vi "GPS-Read.vi"(3 "Organised Output from the GPS":T1(tab)) -> ()   [LabVIEW 2019]
uses:
  <vilib>/Platform/TimedLoop/XDataNode/timing_clust.ctl
  <vilib>/Platform/TimedLoop/XDataNode/nitl_modes.ctl
  <vilib>/Platform/TimedLoop/XDataNode/wakeup.ctl
  <vilib>/Instr/_visa.llb/VISA Configure Serial Port (Instr).vi
  <vilib>/platform/TimedLoop/XDataNode/XDataNode.xnode
  <vilib>/Platform/TimedLoop/XDataNode/XDNodeRunTimeDep.lvlib
panel:
  out "Iteration Duration (ms)":i64
  out "GPGSV":string
  out "number of message":string
  out "msg1":string
  out "Satelite in view":string
  in  "Satelite_id/elevation/azimuth/SNR":enum32{"Msg 1", "Msg 2", "Msg 3", "Msg 4"}(tab)
  out "Satelite_id/elevation/azimuth/SNR":string[](array[string])
  out "Satelite_id/elevation/azimuth/SNR 2":string[](array[string])
  out "Satelite_id/elevation/azimuth/SNR 3":string[](array[string])
  out "Satelite_id/elevation/azimuth/SNR 4":string[](array[string])
  out "Signal ID / Check sum":string[](array[string])
  out "Signal ID / Check sum 2":string[](array[string])
  out "Satelite_id/elevation/azimuth/SNR 8":string[](array[string])
  out "Satelite_id/elevation/azimuth/SNR 7":string[](array[string])
  out "Satelite_id/elevation/azimuth/SNR 6":string[](array[string])
  out "Satelite_id/elevation/azimuth/SNR 5":string[](array[string])
  out "Signal ID / Check sum 3":string[](array[string])
  out "Satelite_id/elevation/azimuth/SNR 12":string[](array[string])
  out "Satelite_id/elevation/azimuth/SNR 11":string[](array[string])
  out "Satelite_id/elevation/azimuth/SNR 10":string[](array[string])
  out "Satelite_id/elevation/azimuth/SNR 9":string[](array[string])
  out "Signal ID / Check sum 4":string[](array[string])
  out "Satelite_id/elevation/azimuth/SNR 16":string[](array[string])
  out "Satelite_id/elevation/azimuth/SNR 15":string[](array[string])
  out "Satelite_id/elevation/azimuth/SNR 14":string[](array[string])
  out "Satelite_id/elevation/azimuth/SNR 13":string[](array[string])
  out "GLGSV 2":string
  out "number of message 2":string
  out "msg1 2":string
  out "Satelite in view 2":string
  in  "Satelite_id/elevation/azimuth/SNR":enum32{"Msg 1", "Msg 2", "Msg 3", "Msg 4"}(tab)
  out "Satelite_id/elevation/azimuth/SNR 20":string[](array[string])
  out "Satelite_id/elevation/azimuth/SNR 19":string[](array[string])
  out "Satelite_id/elevation/azimuth/SNR 18":string[](array[string])
  out "Satelite_id/elevation/azimuth/SNR 17":string[](array[string])
  out "Signal ID / Check sum 5":string[](array[string])
  out "Signal ID / Check sum 6":string[](array[string])
  out "Satelite_id/elevation/azimuth/SNR 21":string[](array[string])
  out "Satelite_id/elevation/azimuth/SNR 22":string[](array[string])
  out "Satelite_id/elevation/azimuth/SNR 23":string[](array[string])
  out "Satelite_id/elevation/azimuth/SNR 24":string[](array[string])
  out "Signal ID / Check sum 7":string[](array[string])
  out "Satelite_id/elevation/azimuth/SNR 25":string[](array[string])
  out "Satelite_id/elevation/azimuth/SNR 26":string[](array[string])
  out "Satelite_id/elevation/azimuth/SNR 27":string[](array[string])
  out "Satelite_id/elevation/azimuth/SNR 28":string[](array[string])
  out "Signal ID / Check sum 8":string[](array[string])
  out "Satelite_id/elevation/azimuth/SNR 29":string[](array[string])
  out "Satelite_id/elevation/azimuth/SNR 30":string[](array[string])
  out "Satelite_id/elevation/azimuth/SNR 31":string[](array[string])
  out "Satelite_id/elevation/azimuth/SNR 32":string[](array[string])
  out "GAGSV 3":string
  out "number of message 3":string
  out "msg1 3":string
  out "Satelite in view 3":string
  in  "Satelite_id/elevation/azimuth/SNR":enum32{"Msg 1", "Msg 2", "Msg 3", "Msg 4"}(tab)
  out "Satelite_id/elevation/azimuth/SNR 37":string[](array[string])
  out "Satelite_id/elevation/azimuth/SNR 36":string[](array[string])
  out "Satelite_id/elevation/azimuth/SNR 35":string[](array[string])
  out "Satelite_id/elevation/azimuth/SNR 34":string[](array[string])
  out "Signal ID / Check sum 9":string[](array[string])
  out "Signal ID / Check sum 10":string[](array[string])
  out "Satelite_id/elevation/azimuth/SNR 38":string[](array[string])
  out "Satelite_id/elevation/azimuth/SNR 39":string[](array[string])
  out "Satelite_id/elevation/azimuth/SNR 40":string[](array[string])
  out "Satelite_id/elevation/azimuth/SNR 41":string[](array[string])
  out "Signal ID / Check sum 11":string[](array[string])
  out "Satelite_id/elevation/azimuth/SNR 42":string[](array[string])
  out "Satelite_id/elevation/azimuth/SNR 43":string[](array[string])
  out "Satelite_id/elevation/azimuth/SNR 44":string[](array[string])
  out "Satelite_id/elevation/azimuth/SNR 45":string[](array[string])
  out "Signal ID / Check sum 12":string[](array[string])
  out "Satelite_id/elevation/azimuth/SNR 46":string[](array[string])
  out "Satelite_id/elevation/azimuth/SNR 47":string[](array[string])
  out "Satelite_id/elevation/azimuth/SNR 48":string[](array[string])
  out "Satelite_id/elevation/azimuth/SNR 49":string[](array[string])
  out "GBGSV 4":string
  out "number of message 4":string
  out "msg1 4":string
  out "Satelite in view 4":string
  in  "Satelite_id/elevation/azimuth/SNR":enum32{"Msg 1", "Msg 2", "Msg 3", "Msg 4"}(tab)
  out "Satelite_id/elevation/azimuth/SNR 54":string[](array[string])
  out "Satelite_id/elevation/azimuth/SNR 53":string[](array[string])
  out "Satelite_id/elevation/azimuth/SNR 52":string[](array[string])
  out "Satelite_id/elevation/azimuth/SNR 51":string[](array[string])
  out "Signal ID / Check sum 13":string[](array[string])
  out "Signal ID / Check sum 14":string[](array[string])
  out "Satelite_id/elevation/azimuth/SNR 55":string[](array[string])
  out "Satelite_id/elevation/azimuth/SNR 56":string[](array[string])
  out "Satelite_id/elevation/azimuth/SNR 57":string[](array[string])
  out "Satelite_id/elevation/azimuth/SNR 58":string[](array[string])
  out "Signal ID / Check sum 15":string[](array[string])
  out "Satelite_id/elevation/azimuth/SNR 59":string[](array[string])
  out "Satelite_id/elevation/azimuth/SNR 60":string[](array[string])
  out "Satelite_id/elevation/azimuth/SNR 61":string[](array[string])
  out "Satelite_id/elevation/azimuth/SNR 62":string[](array[string])
  out "Signal ID / Check sum 16":string[](array[string])
  out "Satelite_id/elevation/azimuth/SNR 63":string[](array[string])
  out "Satelite_id/elevation/azimuth/SNR 64":string[](array[string])
  out "Satelite_id/elevation/azimuth/SNR 65":string[](array[string])
  out "Satelite_id/elevation/azimuth/SNR 66":string[](array[string])
  out "UTC Time":string
  out "N/S":string
  out "Long":string
  out "Mode":string
  out "Status":string
  out "Lat":string
  out "Course over Ground [Degrees]":string
  out "date[ddmmyy]":string
  out "E/W":string
  out "Speed over ground[knot]":string
  out "xxRMC":string
  out "NavStatus":string
  out "Checksum":string
  out "Carriage return":string
  out "Lat":string
  out "NS":string
  out "GLL":string
  out "Long 3":string
  out "EW":string
  out "Time":string
  out "Status 2":string
  out "Positioning mod":string
  out "Check sum":string
  out "Carriage return 2":string
  out "VTG":string
  out "Course over Ground":string
  out "Reference":string
  out "Course over Ground (Magnetic)":string
  out "Reference2":string
  out "Speedover Ground (knots)":string
  out "Units1":string
  out "Speed over ground kph":string
  out "Units 2":string
  out "Position Mode 2":string
  out "Check sum":string
  out "GGA 3":string
  out "UTC time":string
  out "Lat 2":string
  out "NS":string
  out "Long 2":string
  out "EW":string
  out "Pos_indicator":string
  out "Number of Satelite_used":string
  out "hdop":string
  out "msl_altitude":string
  out "altitude_units":string
  out "geoidal_Seperation":string
  out "Separation unit":string
  out "age of Diff corr":string
  out "diffStating":string
  out "Checksum":string
  out "GSA":string
  out "Operation Mode":string
  out "Navigation mode":string
  out "satelite used channel 1":string
  out "satelite used channel 3":string
  out "satelite used channel 4":string
  out "satelite used channel 5":string
  out "satelite used channel 6":string
  out "satelite used channel 7":string
  out "satelite used channel 8":string
  out "satelite used channel 9":string
  out "satelite used channel 10":string
  out "satelite used channel 11":string
  out "satelite used channel 12":string
  out "pdop":string
  out "hdop 2":string
  out "vdop":string
  out "System ID":string
  out "Checksum":string
  out "satelite used channel 2":string
  out "Raw output from GPS":string
  in  "stop":bool
  # "Signal ID / Check sum"
  # "Signal ID / Check sum"
  # "Signal ID / Check sum"
  # "Signal ID / Check sum"
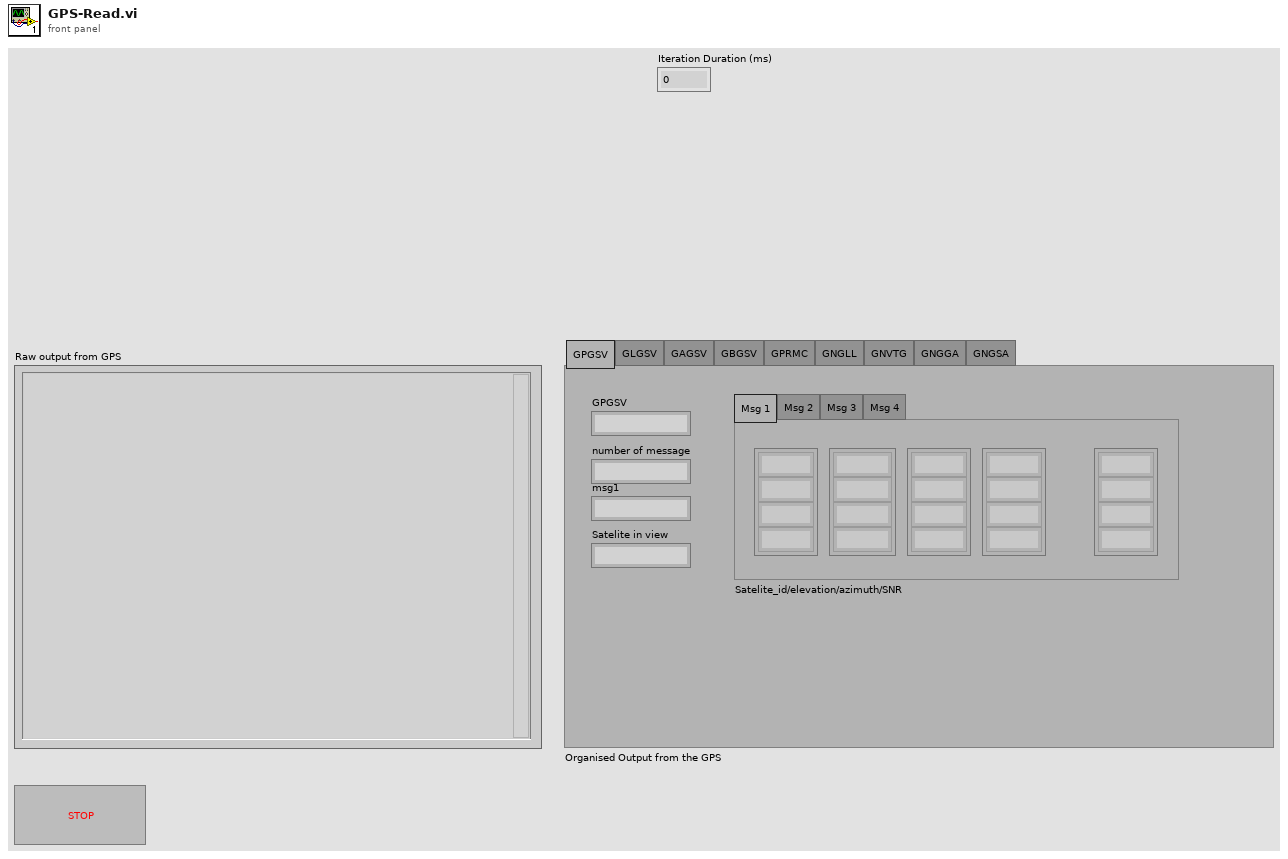
[diagram p1: front panel]
types:
  T1 = enum32{"GPGSV", "GLGSV", "GAGSV", "GBGSV", "GPRMC", "GNGLL", "GNVTG", "GNGGA", "GNGSA"}
  T2 = typedef "XDNodeRunTimeDep.lvlib/timing_clust.ctl" = cluster{"Expected End [f-1]":u64, "Actual End [f-1]":u64, "Finished Late? [f-1]":bool, "Expected End [i-1]":u64, "Actual End [i-1]":u64, "Finished Late? [i-1]":bool, "Expected Start [i]":u64, "Actual Start [i]":u64, "Expected Start [f]":u64, "Actual Start [f]":u64, "Source Name":string, "Structure Name":string, "Period":i64, "Deadline":i64, "Offset":i64, "Start":i64, "Priority":i32, "Timeout":i32, "Mode":T3, "Wakeup Reason":T4, "Error":errorcluster, "Source Type":string, "Secondary Source Type":string, "Global End Time":u64, "Global Start Time":u64, "Frame Duration":u64, "Iteration Duration":u64, "Assigned CPU":i32, "I/O Scan Engine Mode":u32}
  T3 = typedef "XDNodeRunTimeDep.lvlib/nitl_modes.ctl" = enum32{"No Change", "Process missed periods, maintain original phase", "Discard missed periods, maintain original phase", "Process missed periods, ignore original phase", "Discard missed periods, ignore original phase"}
  T4 = typedef "XDNodeRunTimeDep.lvlib/wakeup.ctl" = enum32{"Normal", "Aborted", "Asynchronous wakeup", "Timing source error", "Timed loop error", "Timeout"}
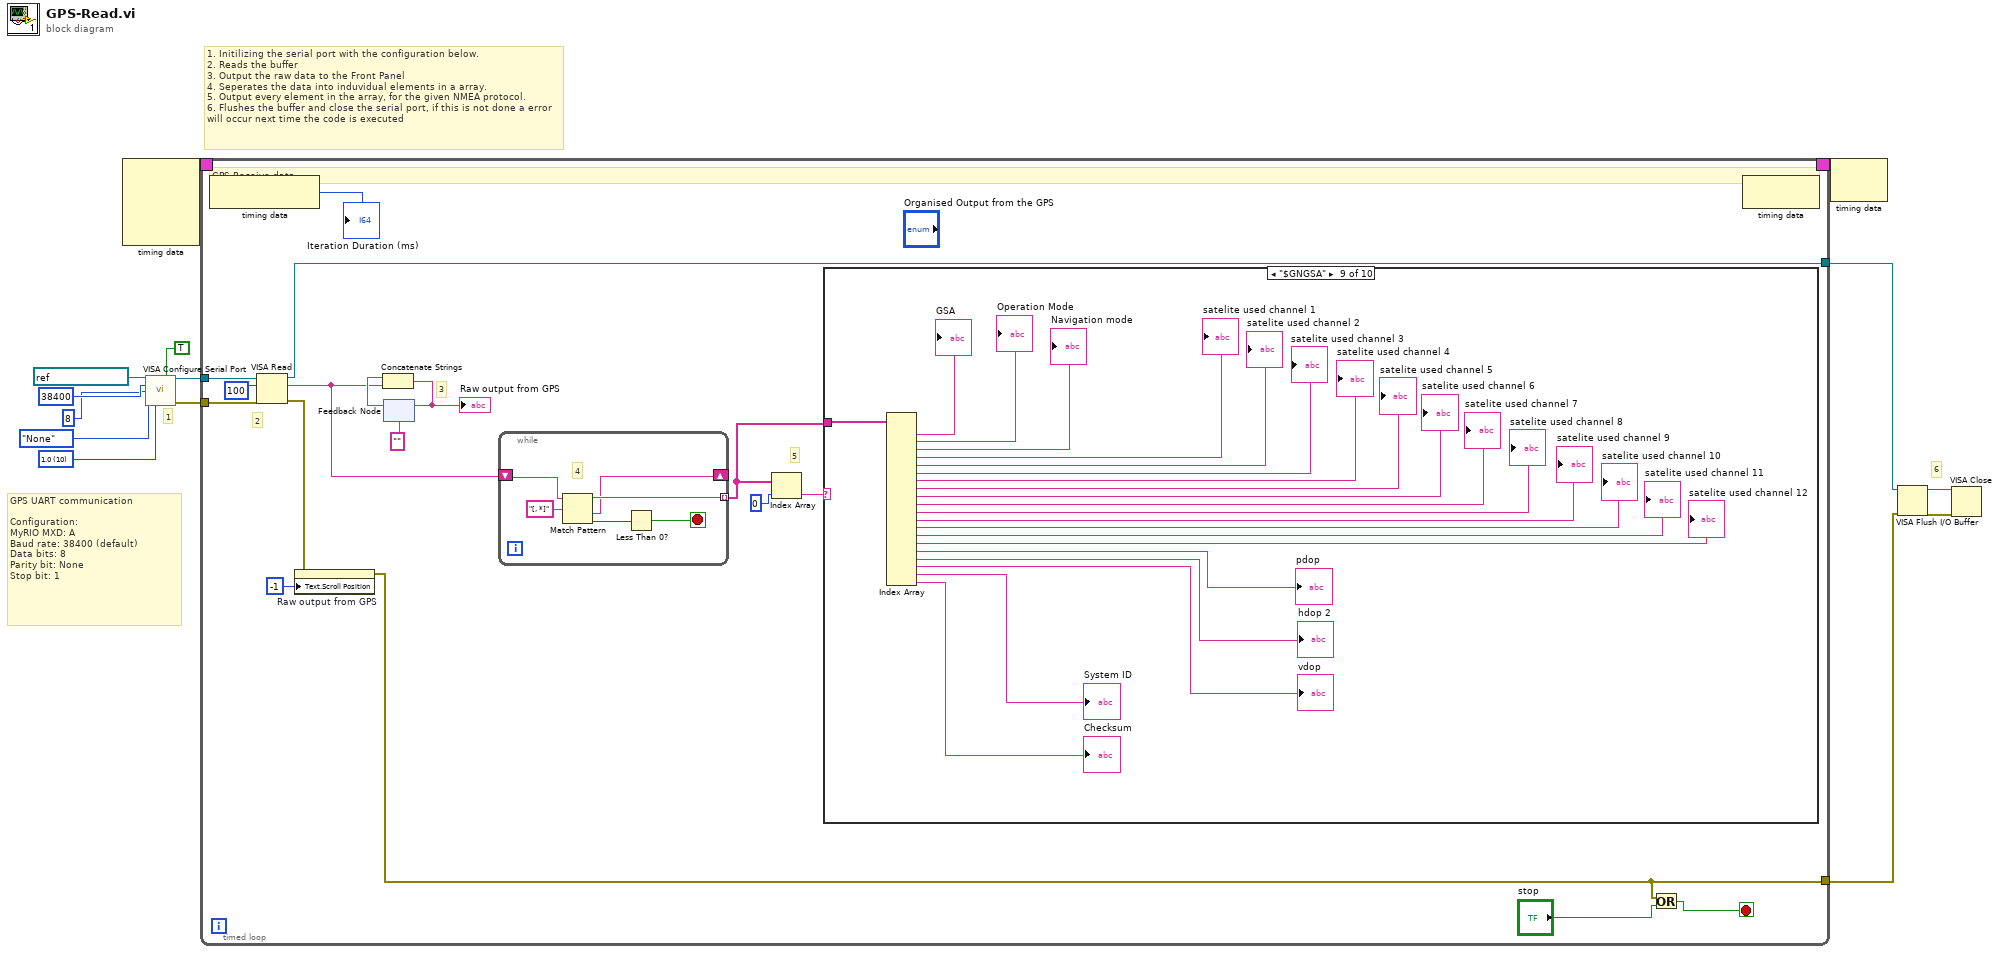
[diagram p0: block diagram]
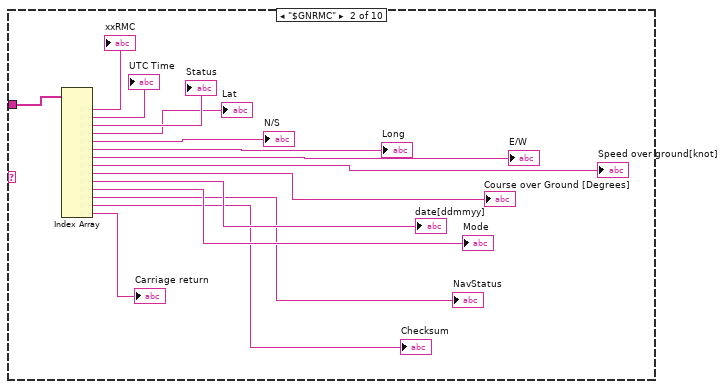
[diagram p3: hidden frame]
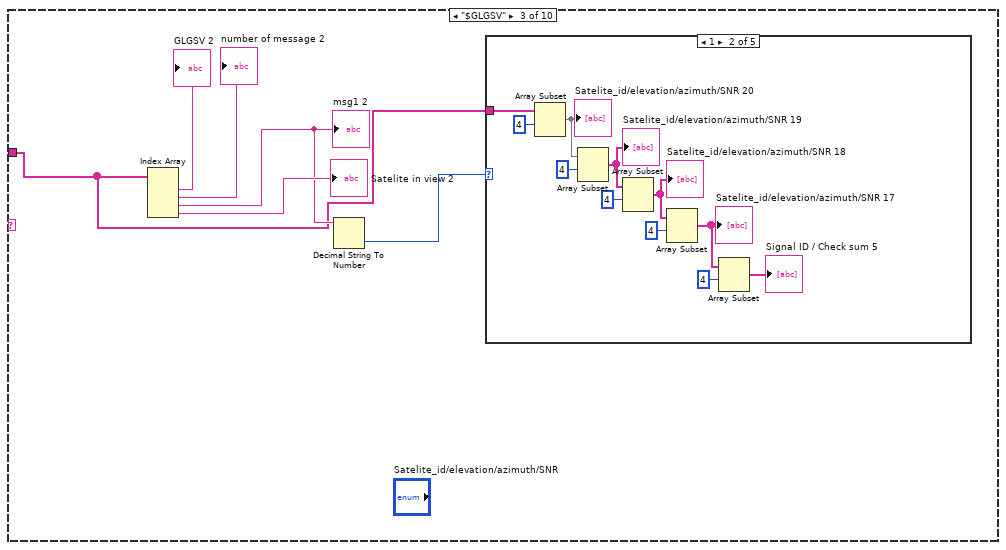
[diagram p4: hidden frame]
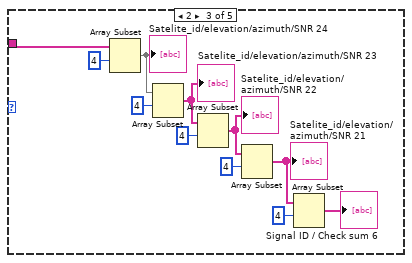
[diagram p6: hidden frame]
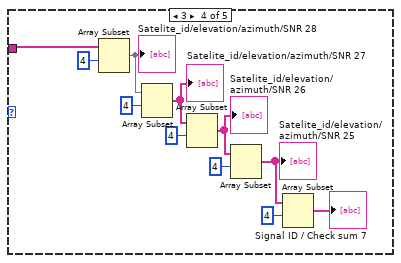
[diagram p7: hidden frame]
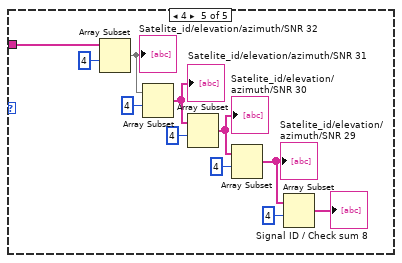
[diagram p8: hidden frame]
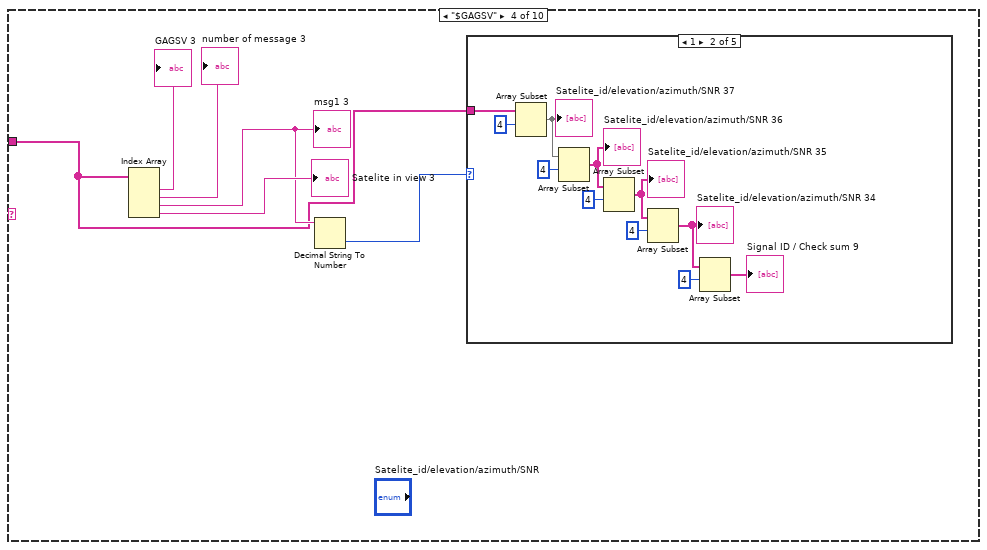
[diagram p9: hidden frame]
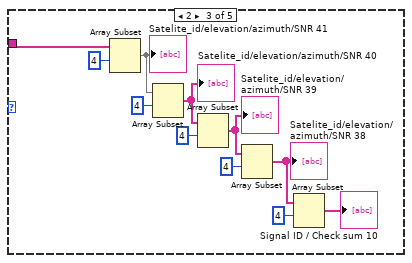
[diagram p11: hidden frame]
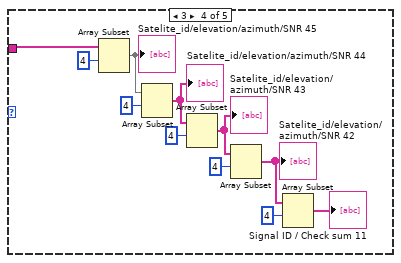
[diagram p12: hidden frame]
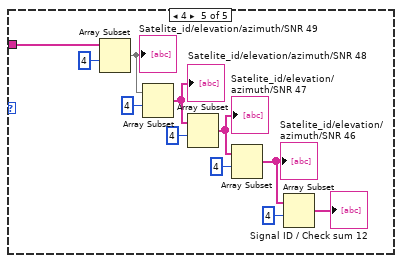
[diagram p13: hidden frame]
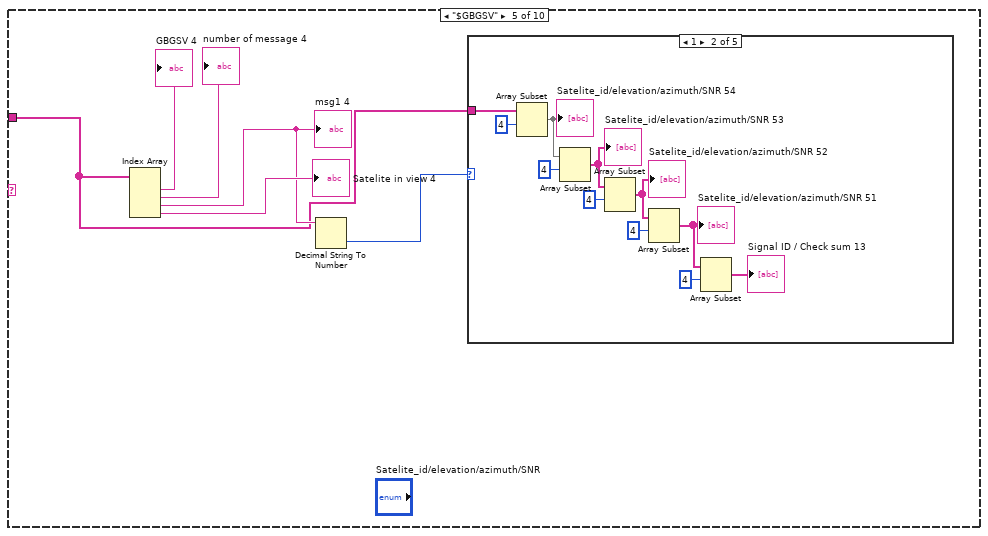
[diagram p14: hidden frame]
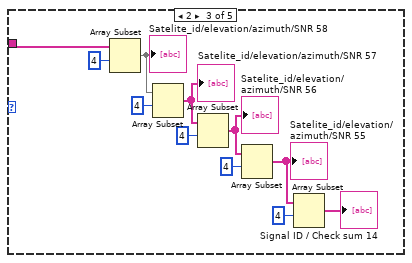
[diagram p16: hidden frame]
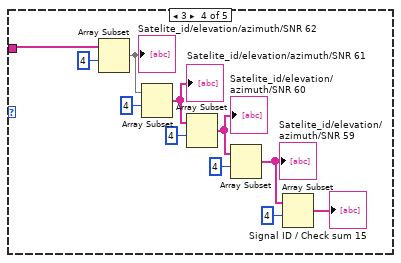
[diagram p17: hidden frame]
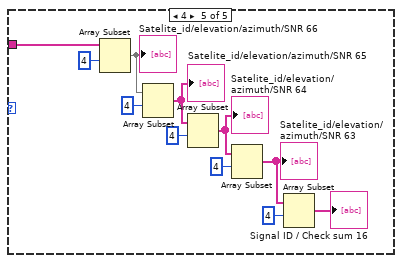
[diagram p18: hidden frame]
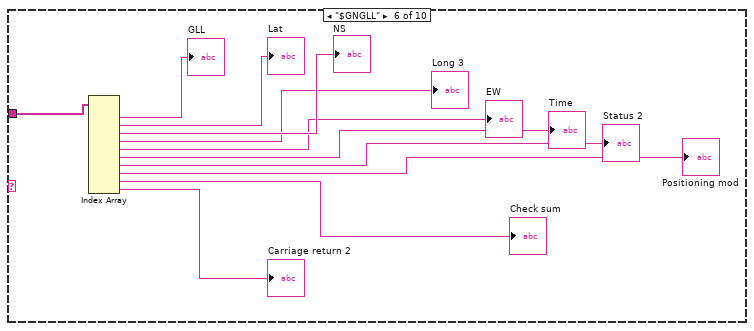
[diagram p19: hidden frame]
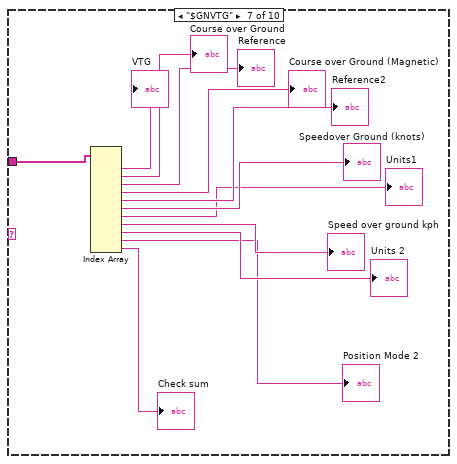
[diagram p20: hidden frame]
diagram:
  w9 = u16 10 items=["1.0"=10, "1.5"=15, "2.0"=20] ("stop bits (10: 1 bit)")
  # "6"
  # "1"
  # "1. Initilizing the serial port with the configuration below.\n2. Reads the buffer\n3. Output the raw data to the Front Panel\n4. Seperates the data into induvidual elements in a array.\n5. Output every element in the array, for the given NMEA protocol.\n6. Flushes the buffer and close the serial port, if this is not done a error will occur next time the code is executed"
  # "GPS UART communication\n\nConfiguration:\nMyRIO MXD: A\nBaud rate: 38400 (default)\nData bits: 8\nParity bit: None\nStop bit: 1"
  n1 = node-c288() -> (w2:T2)  [unwired: 4 in]
  n2 = call-poly "VISA Configure Serial Port"("VISA resource name"=refnum<visa-resource-name> "ASRL1::INSTR", "Enable Termination\nChar (T)"=TRUE ("Enable Termination\nChar (T)"), "baud rate (9600)"=u32 38400, "data bits (8)"=u16 8, "parity (0:none)"=enum16{"None", "Odd", "Even", "Mark", "Space"}."None", "stop bits (10: 1 bit)"=w9) -> ("VISA resource name out"=w5:refnum<visa-resource-name>, "error out"=w4:errorcluster)  [unwired: 8 in]
  n3 = timed-loop {
    tunnel: [w23] -> w6
    tunnel: w5 -> [w22]
    tunnel: w4 -> [w21]
    tunnel: [w17] -> w3
    timing: w2 -> [_]
    timing-out: [_] -> w1
    stop <- w20 stop-if-true
    # "5"
    # "3"
    # "2"
    # "GPS Receive data"
    n4 = node-c288() -> (→"Iteration Duration (ms)":i64)  [unwired: 1 in]
    n5 = VISA Read(VISA resource name=w22, byte count=u32 100, error in (no error)=w21) -> (VISA resource name out=w23:refnum<visa-resource-name>, read buffer=w27:string, error out=w18:errorcluster)  [unwired: 1 out]
    n6 = property on="Raw output from GPS" class="Str"(error in=w18, "Text.Scroll Position"=-1 ("Label.Scroll Position")) -> (error out=w17:errorcluster)  [unwired: 1 in, 1 out]
    n7 = feedback #1("") -> (w29:string)
    n8 = Concatenate Strings(w29, w27) -> (w30:string)
    "Raw output from GPS" <- w30
    n9 = feedback-in #1(w30) -> ()
    n10 = while {
      tunnel: [w314] -> w24 mode=indexing
      shift-right: [w313] -> _
      shift-left: w27 -> [w316]
      stop <- w311 stop-if-true
      # "4"
      n11 = Match Pattern(string=w316, regular expression="[, *]") -> (before substring=w314:string, after substring=w313:string, offset past match=w312:i32)  [unwired: 1 in, 1 out]
      n12 = Less Than 0?(x=w312) -> (x < 0?=w311:bool)
    }
    n13 = Index Array(array=w24, index=0) -> (element=w25:string)
    n14 = case shown="\"$GNGSA\"" w25 {
      tunnel: w24 -> [_ w49 w50 w100 w150 w210 w222 w239 w260 w261]
      frame "False", Default {
      }
      frame "$GNRMC" {
        n15 = Index Array(array=w49) -> (element #1=→"xxRMC":string, element #2=→"UTC Time":string, element #3=→"Status":string, element #4=→"Lat":string, element #5=→"N/S":string, element #6=→"Long":string, element #7=→"E/W":string, element #8=→"Speed over ground[knot]":string, element #9=→"Course over Ground [Degrees]":string, element #10=→"date[ddmmyy]":string, element #11=→"Mode":string, element #12=→"NavStatus":string, element #13=→"Checksum":string, element #14=→"Carriage return":string)  [unwired: 14 in]
      }
      frame "$GLGSV" {
        n16 = Index Array(array=w50) -> (element #1=→"GLGSV 2":string, element #2=→"number of message 2":string, element #3=w52:string, element #4=→"Satelite in view 2":string)  [unwired: 4 in]
        "msg1 2" <- w52
        n17 = Decimal String To Number(string=w52) -> (number=w51:i32)  [unwired: 2 in, 1 out]
        n18 = case shown="1" w51 {
          tunnel: w50 -> [_ w57 w67 w78 w89]
          frame 0, Default {
          }
          frame 1 {
            n19 = Array Subset(array=w57, index=4) -> (w62:string[])  [unwired: 1 in]
            "Satelite_id/elevation/azimuth/SNR 20" <- w62
            n20 = Array Subset(array=w62, index=4) -> (w63:string[])  [unwired: 1 in]
            "Satelite_id/elevation/azimuth/SNR 19" <- w63
            n21 = Array Subset(array=w63, index=4) -> (w64:string[])  [unwired: 1 in]
            "Satelite_id/elevation/azimuth/SNR 18" <- w64
            n22 = Array Subset(array=w64, index=4) -> (w66:string[])  [unwired: 1 in]
            "Satelite_id/elevation/azimuth/SNR 17" <- w66
            n23 = Array Subset(array=w66, index=4) -> (→"Signal ID / Check sum 5":string[])  [unwired: 1 in]
          }
          frame 2 {
            n24 = Array Subset(array=w67, index=4) -> (w73:string[])  [unwired: 1 in]
            "Satelite_id/elevation/azimuth/SNR 24" <- w73
            n25 = Array Subset(array=w73, index=4) -> (w74:string[])  [unwired: 1 in]
            "Satelite_id/elevation/azimuth/SNR 23" <- w74
            n26 = Array Subset(array=w74, index=4) -> (w75:string[])  [unwired: 1 in]
            "Satelite_id/elevation/azimuth/SNR 22" <- w75
            n27 = Array Subset(array=w75, index=4) -> (w77:string[])  [unwired: 1 in]
            "Satelite_id/elevation/azimuth/SNR 21" <- w77
            n28 = Array Subset(array=w77, index=4) -> (→"Signal ID / Check sum 6":string[])  [unwired: 1 in]
          }
          frame 3 {
            n29 = Array Subset(array=w78, index=4) -> (w84:string[])  [unwired: 1 in]
            "Satelite_id/elevation/azimuth/SNR 28" <- w84
            n30 = Array Subset(array=w84, index=4) -> (w85:string[])  [unwired: 1 in]
            "Satelite_id/elevation/azimuth/SNR 27" <- w85
            n31 = Array Subset(array=w85, index=4) -> (w86:string[])  [unwired: 1 in]
            "Satelite_id/elevation/azimuth/SNR 26" <- w86
            n32 = Array Subset(array=w86, index=4) -> (w88:string[])  [unwired: 1 in]
            "Satelite_id/elevation/azimuth/SNR 25" <- w88
            n33 = Array Subset(array=w88, index=4) -> (→"Signal ID / Check sum 7":string[])  [unwired: 1 in]
          }
          frame 4 {
            n34 = Array Subset(array=w89, index=4) -> (w95:string[])  [unwired: 1 in]
            "Satelite_id/elevation/azimuth/SNR 32" <- w95
            n35 = Array Subset(array=w95, index=4) -> (w96:string[])  [unwired: 1 in]
            "Satelite_id/elevation/azimuth/SNR 31" <- w96
            n36 = Array Subset(array=w96, index=4) -> (w97:string[])  [unwired: 1 in]
            "Satelite_id/elevation/azimuth/SNR 30" <- w97
            n37 = Array Subset(array=w97, index=4) -> (w99:string[])  [unwired: 1 in]
            "Satelite_id/elevation/azimuth/SNR 29" <- w99
            n38 = Array Subset(array=w99, index=4) -> (→"Signal ID / Check sum 8":string[])  [unwired: 1 in]
          }
        }
      }
      frame "$GAGSV" {
        n39 = Index Array(array=w100) -> (element #1=→"GAGSV 3":string, element #2=→"number of message 3":string, element #3=w102:string, element #4=→"Satelite in view 3":string)  [unwired: 4 in]
        "msg1 3" <- w102
        n40 = Decimal String To Number(string=w102) -> (number=w101:i32)  [unwired: 2 in, 1 out]
        n41 = case shown="1" w101 {
          tunnel: w100 -> [_ w107 w117 w128 w139]
          frame 0, Default {
          }
          frame 1 {
            n42 = Array Subset(array=w107, index=4) -> (w112:string[])  [unwired: 1 in]
            "Satelite_id/elevation/azimuth/SNR 37" <- w112
            n43 = Array Subset(array=w112, index=4) -> (w113:string[])  [unwired: 1 in]
            "Satelite_id/elevation/azimuth/SNR 36" <- w113
            n44 = Array Subset(array=w113, index=4) -> (w114:string[])  [unwired: 1 in]
            "Satelite_id/elevation/azimuth/SNR 35" <- w114
            n45 = Array Subset(array=w114, index=4) -> (w116:string[])  [unwired: 1 in]
            "Satelite_id/elevation/azimuth/SNR 34" <- w116
            n46 = Array Subset(array=w116, index=4) -> (→"Signal ID / Check sum 9":string[])  [unwired: 1 in]
          }
          frame 2 {
            n47 = Array Subset(array=w117, index=4) -> (w123:string[])  [unwired: 1 in]
            "Satelite_id/elevation/azimuth/SNR 41" <- w123
            n48 = Array Subset(array=w123, index=4) -> (w124:string[])  [unwired: 1 in]
            "Satelite_id/elevation/azimuth/SNR 40" <- w124
            n49 = Array Subset(array=w124, index=4) -> (w125:string[])  [unwired: 1 in]
            "Satelite_id/elevation/azimuth/SNR 39" <- w125
            n50 = Array Subset(array=w125, index=4) -> (w127:string[])  [unwired: 1 in]
            "Satelite_id/elevation/azimuth/SNR 38" <- w127
            n51 = Array Subset(array=w127, index=4) -> (→"Signal ID / Check sum 10":string[])  [unwired: 1 in]
          }
          frame 3 {
            n52 = Array Subset(array=w128, index=4) -> (w134:string[])  [unwired: 1 in]
            "Satelite_id/elevation/azimuth/SNR 45" <- w134
            n53 = Array Subset(array=w134, index=4) -> (w135:string[])  [unwired: 1 in]
            "Satelite_id/elevation/azimuth/SNR 44" <- w135
            n54 = Array Subset(array=w135, index=4) -> (w136:string[])  [unwired: 1 in]
            "Satelite_id/elevation/azimuth/SNR 43" <- w136
            n55 = Array Subset(array=w136, index=4) -> (w138:string[])  [unwired: 1 in]
            "Satelite_id/elevation/azimuth/SNR 42" <- w138
            n56 = Array Subset(array=w138, index=4) -> (→"Signal ID / Check sum 11":string[])  [unwired: 1 in]
          }
          frame 4 {
            n57 = Array Subset(array=w139, index=4) -> (w145:string[])  [unwired: 1 in]
            "Satelite_id/elevation/azimuth/SNR 49" <- w145
            n58 = Array Subset(array=w145, index=4) -> (w146:string[])  [unwired: 1 in]
            "Satelite_id/elevation/azimuth/SNR 48" <- w146
            n59 = Array Subset(array=w146, index=4) -> (w147:string[])  [unwired: 1 in]
            "Satelite_id/elevation/azimuth/SNR 47" <- w147
            n60 = Array Subset(array=w147, index=4) -> (w149:string[])  [unwired: 1 in]
            "Satelite_id/elevation/azimuth/SNR 46" <- w149
            n61 = Array Subset(array=w149, index=4) -> (→"Signal ID / Check sum 12":string[])  [unwired: 1 in]
          }
        }
      }
      frame "$GBGSV" {
        n62 = Index Array(array=w150) -> (element #1=→"GBGSV 4":string, element #2=→"number of message 4":string, element #3=w152:string, element #4=→"Satelite in view 4":string)  [unwired: 4 in]
        "msg1 4" <- w152
        n63 = Decimal String To Number(string=w152) -> (number=w151:i32)  [unwired: 2 in, 1 out]
        n64 = case shown="1" w151 {
          tunnel: w150 -> [_ w157 w167 w178 w189]
          frame 0, Default {
          }
          frame 1 {
            n65 = Array Subset(array=w157, index=4) -> (w162:string[])  [unwired: 1 in]
            "Satelite_id/elevation/azimuth/SNR 54" <- w162
            n66 = Array Subset(array=w162, index=4) -> (w163:string[])  [unwired: 1 in]
            "Satelite_id/elevation/azimuth/SNR 53" <- w163
            n67 = Array Subset(array=w163, index=4) -> (w164:string[])  [unwired: 1 in]
            "Satelite_id/elevation/azimuth/SNR 52" <- w164
            n68 = Array Subset(array=w164, index=4) -> (w166:string[])  [unwired: 1 in]
            "Satelite_id/elevation/azimuth/SNR 51" <- w166
            n69 = Array Subset(array=w166, index=4) -> (→"Signal ID / Check sum 13":string[])  [unwired: 1 in]
          }
          frame 2 {
            n70 = Array Subset(array=w167, index=4) -> (w173:string[])  [unwired: 1 in]
            "Satelite_id/elevation/azimuth/SNR 58" <- w173
            n71 = Array Subset(array=w173, index=4) -> (w174:string[])  [unwired: 1 in]
            "Satelite_id/elevation/azimuth/SNR 57" <- w174
            n72 = Array Subset(array=w174, index=4) -> (w175:string[])  [unwired: 1 in]
            "Satelite_id/elevation/azimuth/SNR 56" <- w175
            n73 = Array Subset(array=w175, index=4) -> (w177:string[])  [unwired: 1 in]
            "Satelite_id/elevation/azimuth/SNR 55" <- w177
            n74 = Array Subset(array=w177, index=4) -> (→"Signal ID / Check sum 14":string[])  [unwired: 1 in]
          }
          frame 3 {
            n75 = Array Subset(array=w178, index=4) -> (w184:string[])  [unwired: 1 in]
            "Satelite_id/elevation/azimuth/SNR 62" <- w184
            n76 = Array Subset(array=w184, index=4) -> (w185:string[])  [unwired: 1 in]
            "Satelite_id/elevation/azimuth/SNR 61" <- w185
            n77 = Array Subset(array=w185, index=4) -> (w186:string[])  [unwired: 1 in]
            "Satelite_id/elevation/azimuth/SNR 60" <- w186
            n78 = Array Subset(array=w186, index=4) -> (w188:string[])  [unwired: 1 in]
            "Satelite_id/elevation/azimuth/SNR 59" <- w188
            n79 = Array Subset(array=w188, index=4) -> (→"Signal ID / Check sum 15":string[])  [unwired: 1 in]
          }
          frame 4 {
            n80 = Array Subset(array=w189, index=4) -> (w195:string[])  [unwired: 1 in]
            "Satelite_id/elevation/azimuth/SNR 66" <- w195
            n81 = Array Subset(array=w195, index=4) -> (w196:string[])  [unwired: 1 in]
            "Satelite_id/elevation/azimuth/SNR 65" <- w196
            n82 = Array Subset(array=w196, index=4) -> (w197:string[])  [unwired: 1 in]
            "Satelite_id/elevation/azimuth/SNR 64" <- w197
            n83 = Array Subset(array=w197, index=4) -> (w199:string[])  [unwired: 1 in]
            "Satelite_id/elevation/azimuth/SNR 63" <- w199
            n84 = Array Subset(array=w199, index=4) -> (→"Signal ID / Check sum 16":string[])  [unwired: 1 in]
          }
        }
      }
      frame "$GNGLL" {
        n85 = Index Array(array=w210) -> (element #1=→"GLL":string, element #2=→"Lat":string, element #3=→"NS":string, element #4=→"Long 3":string, element #5=→"EW":string, element #6=→"Time":string, element #7=→"Status 2":string, element #8=→"Positioning mod":string, element #9=→"Check sum":string, element #10=→"Carriage return 2":string)  [unwired: 10 in]
      }
      frame "$GNVTG" {
        n86 = Index Array(array=w222) -> (element #1=→"VTG":string, element #2=→"Course over Ground":string, element #3=→"Reference":string, element #4=→"Course over Ground (Magnetic)":string, element #5=→"Reference2":string, element #6=→"Speedover Ground (knots)":string, element #7=→"Units1":string, element #8=→"Speed over ground kph":string, element #9=→"Units 2":string, element #10=→"Position Mode 2":string, element #11=→"Check sum":string)  [unwired: 11 in]
      }
      frame "$GNGGA" {
        n87 = Index Array(array=w239) -> (element #1=→"GGA 3":string, element #2=→"UTC time":string, element #3=→"Lat 2":string, element #4=→"NS":string, element #5=→"Long 2":string, element #6=→"EW":string, element #7=→"Pos_indicator":string, element #8=→"Number of Satelite_used":string, element #9=→"hdop":string, element #10=→"msl_altitude":string, element #11=→"altitude_units":string, element #12=→"geoidal_Seperation":string, element #13=→"Separation unit":string, element #14=→"age of Diff corr":string, element #15=→"diffStating":string, element #16=→"Checksum":string)  [unwired: 16 in]
      }
      frame "$GNGSA" {
        n88 = Index Array(array=w260) -> (element #1=→"GSA":string, element #2=→"Operation Mode":string, element #3=→"Navigation mode":string, element #4=→"satelite used channel 1":string, element #5=→"satelite used channel 2":string, element #6=→"satelite used channel 3":string, element #7=→"satelite used channel 4":string, element #8=→"satelite used channel 5":string, element #9=→"satelite used channel 6":string, element #10=→"satelite used channel 7":string, element #11=→"satelite used channel 8":string, element #12=→"satelite used channel 9":string, element #13=→"satelite used channel 10":string, element #14=→"satelite used channel 11":string, element #15=→"satelite used channel 12":string, element #16=→"pdop":string, element #17=→"hdop 2":string, element #18=→"vdop":string, element #19=→"System ID":string, element #20=→"Checksum":string)  [unwired: 20 in]
      }
      frame "$GPGSV" {
        n89 = Index Array(array=w261) -> (element #1=→"GPGSV":string, element #2=→"number of message":string, element #3=w263:string, element #4=→"Satelite in view":string)  [unwired: 4 in]
        "msg1" <- w263
        n90 = Decimal String To Number(string=w263) -> (number=w262:i32)  [unwired: 2 in, 1 out]
        n91 = case shown="1" w262 {
          tunnel: w261 -> [_ w268 w278 w289 w300]
          frame 0, Default {
          }
          frame 1 {
            n92 = Array Subset(array=w268, index=4) -> (w273:string[])  [unwired: 1 in]
            "Satelite_id/elevation/azimuth/SNR" <- w273
            n93 = Array Subset(array=w273, index=4) -> (w274:string[])  [unwired: 1 in]
            "Satelite_id/elevation/azimuth/SNR 2" <- w274
            n94 = Array Subset(array=w274, index=4) -> (w275:string[])  [unwired: 1 in]
            "Satelite_id/elevation/azimuth/SNR 3" <- w275
            n95 = Array Subset(array=w275, index=4) -> (w277:string[])  [unwired: 1 in]
            "Satelite_id/elevation/azimuth/SNR 4" <- w277
            n96 = Array Subset(array=w277, index=4) -> (→"Signal ID / Check sum":string[])  [unwired: 1 in]
          }
          frame 2 {
            n97 = Array Subset(array=w278, index=4) -> (w284:string[])  [unwired: 1 in]
            "Satelite_id/elevation/azimuth/SNR 5" <- w284
            n98 = Array Subset(array=w284, index=4) -> (w285:string[])  [unwired: 1 in]
            "Satelite_id/elevation/azimuth/SNR 6" <- w285
            n99 = Array Subset(array=w285, index=4) -> (w286:string[])  [unwired: 1 in]
            "Satelite_id/elevation/azimuth/SNR 7" <- w286
            n100 = Array Subset(array=w286, index=4) -> (w288:string[])  [unwired: 1 in]
            "Satelite_id/elevation/azimuth/SNR 8" <- w288
            n101 = Array Subset(array=w288, index=4) -> (→"Signal ID / Check sum 2":string[])  [unwired: 1 in]
          }
          frame 3 {
            n102 = Array Subset(array=w289, index=4) -> (w295:string[])  [unwired: 1 in]
            "Satelite_id/elevation/azimuth/SNR 9" <- w295
            n103 = Array Subset(array=w295, index=4) -> (w296:string[])  [unwired: 1 in]
            "Satelite_id/elevation/azimuth/SNR 10" <- w296
            n104 = Array Subset(array=w296, index=4) -> (w297:string[])  [unwired: 1 in]
            "Satelite_id/elevation/azimuth/SNR 11" <- w297
            n105 = Array Subset(array=w297, index=4) -> (w299:string[])  [unwired: 1 in]
            "Satelite_id/elevation/azimuth/SNR 12" <- w299
            n106 = Array Subset(array=w299, index=4) -> (→"Signal ID / Check sum 3":string[])  [unwired: 1 in]
          }
          frame 4 {
            n107 = Array Subset(array=w300, index=4) -> (w306:string[])  [unwired: 1 in]
            "Satelite_id/elevation/azimuth/SNR 13" <- w306
            n108 = Array Subset(array=w306, index=4) -> (w307:string[])  [unwired: 1 in]
            "Satelite_id/elevation/azimuth/SNR 14" <- w307
            n109 = Array Subset(array=w307, index=4) -> (w308:string[])  [unwired: 1 in]
            "Satelite_id/elevation/azimuth/SNR 15" <- w308
            n110 = Array Subset(array=w308, index=4) -> (w310:string[])  [unwired: 1 in]
            "Satelite_id/elevation/azimuth/SNR 16" <- w310
            n111 = Array Subset(array=w310, index=4) -> (→"Signal ID / Check sum 4":string[])  [unwired: 1 in]
          }
        }
      }
    }
    n112 = Or(x=w17, y="stop") -> (x .or. y?=w20:bool)
    n113 = node-c288() -> ()  [unwired: 1 in, 1 out]
  }
  n114 = node-c288(w1) -> ()  [unwired: 1 out]
  n115 = VISA Flush I/O Buffer(VISA resource name=w6, error in (no error)=w3) -> (VISA resource name out=w8:refnum<visa-resource-name>, error out=w7:errorcluster)  [unwired: 1 in]
  n116 = VISA Close(VISA resource name=w8, error in (no error)=w7) -> ()  [unwired: 1 out]
